vi "setRoots.vi"(8 "error in (no error)":errorcluster, 10 "Roots":refnum<data-value>[](array[refnum]), 11 "MultiTree in":refnum<class "MultiTree.lvclass">) -> (0 "error out":errorcluster, 3 "MultiTree out":refnum<class "MultiTree.lvclass">)   [LabVIEW 2014, in "MultiTree.lvlib" / "MultiTree.lvclass"]
uses:
  <userlib>/AdvancedDataStructures/ClassBased/MultiTree/MultiTree.lvclass
  <userlib>/AdvancedDataStructures/ClassBased/MultiTreeNode/MultiTreeNode.lvclass
  <userlib>/AdvancedDataStructures/ClassBased/MultiTree/MultiTree.lvclass/MultiTree.ctl
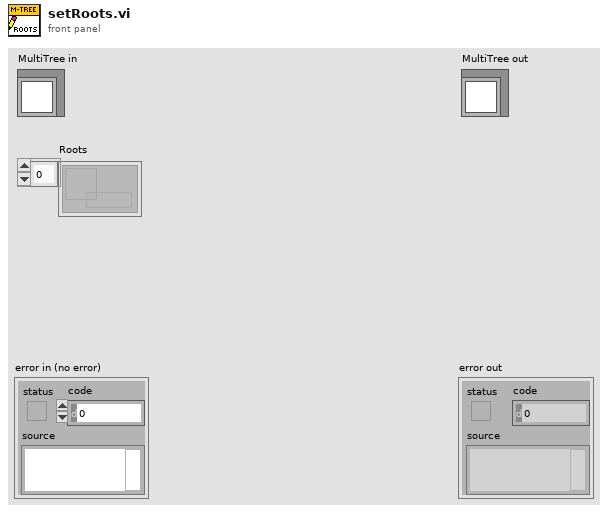
[diagram p1: front panel]
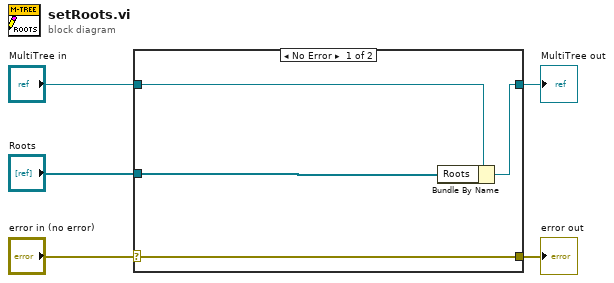
[diagram p0: block diagram]
diagram:
  n1 = case shown="No Error" "error in (no error)" {
    selector: "error in (no error)" -> [w9 w10]
    tunnel: [w9 w10] -> w4
    tunnel: [w7 w11] -> w2
    tunnel: "MultiTree in" -> [w8 w11]
    tunnel: "Roots" -> [w6 _]
    frame No Error {
      n2 = Bundle By Name(cluster=w8, "Roots"=w6) -> (w7:refnum<class "MultiTree.lvclass">)
    }
    frame Error {
    }
  }
  "error out" <- w4
  "MultiTree out" <- w2
